vi "global_variables.vi"() -> ()   [LabVIEW 2010]
uses:
  common/enumerations/config_type_enum.ctl
panel:
  out "running?":bool
  in  "top level configuration registry key":string="HeliosScan"
  in  "config type":T1=enum."global config files"
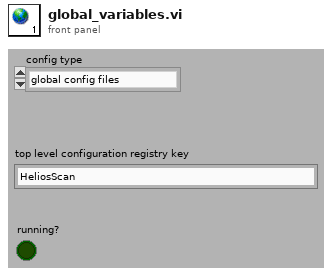
[diagram p1: front panel]
types:
  T1 = typedef "config_type_enum.ctl" = enum16{"local config files", "global config files", "local Windows registry", "global Windows registry"}
diagram:
